vi "File time naming.vi"() -> (3 "result string":string)   [LabVIEW 2018]
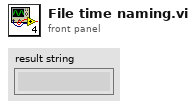
[diagram p1: front panel]
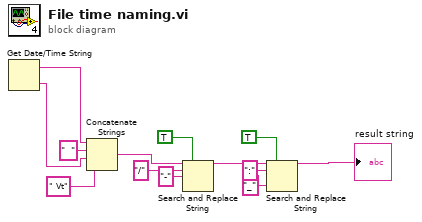
[diagram p0: block diagram]
diagram:
  n1 = Get Date/Time String() -> (date string=w11:string, time string=w12:string)  [unwired: 3 in]
  n2 = Concatenate Strings(w11, "  " ("string"), w12, " Vt" ("string")) -> (w1:string)
  n3 = Search and Replace String(replace all?=TRUE ("replace all? (F)"), input string=w1, search string="/", replace string="-" ("replace string (\"\")")) -> (result string=w5:string)  [unwired: 4 in, 3 out]
  n4 = Search and Replace String(replace all?=TRUE ("replace all? (F)"), input string=w5, search string=":", replace string="_" ("replace string (\"\")")) -> (result string=→"result string":string)  [unwired: 4 in, 3 out]
